vi "MKS_VIs.vi"() -> ()   [LabVIEW 2013]
uses:
  <userlib>/_mks/common/mks setpoint type.ctl
  <userlib>/_mks/common/mks alt status setpoint selection.ctl
  <userlib>/_mks/common/mks valve mode.ctl
  <userlib>/_mks/additional/mks request gain A (46).vi
  <userlib>/_mks/additional/mks request lead A value (41).vi
  <userlib>/_mks/additional/mks request analog setpoint type (25).vi
  <userlib>/_mks/additional/mks request setpoint analog value (0).vi
  <userlib>/_mks/additional/mks request softstart rate analog value (20).vi
  <userlib>/_mks/additional/mks request low threshold 1 (11).vi
panel:
  in  "stop":bool
  in  "valve mode":T1
  in  "setpoint value":dbl min=0.0 max=100.0 format="%.2g"
  in  "setpoint type":T2
  in  "setpoint selection":T3=enum."setpoint A"
  out "setpoint":dbl format="%.3g"
  out "setpoint type":T2
  out "error out":errorcluster
  out "Pressure (Torr)":dbl
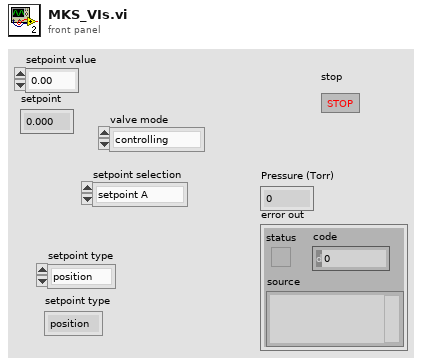
[diagram p1: front panel]
types:
  T1 = typedef "mks valve mode.ctl" = enum16{"controlling", "hold", "valve open", "unknoen", "valve close"}
  T2 = typedef "mks setpoint type.ctl" = enum16{"position", "pressure"}
  T3 = typedef "mks alt status setpoint selection.ctl" = enum16{"analog setpoint", "setpoint A", "setpoint B", "setpoint C", "setpoint D", "setpoint E"}
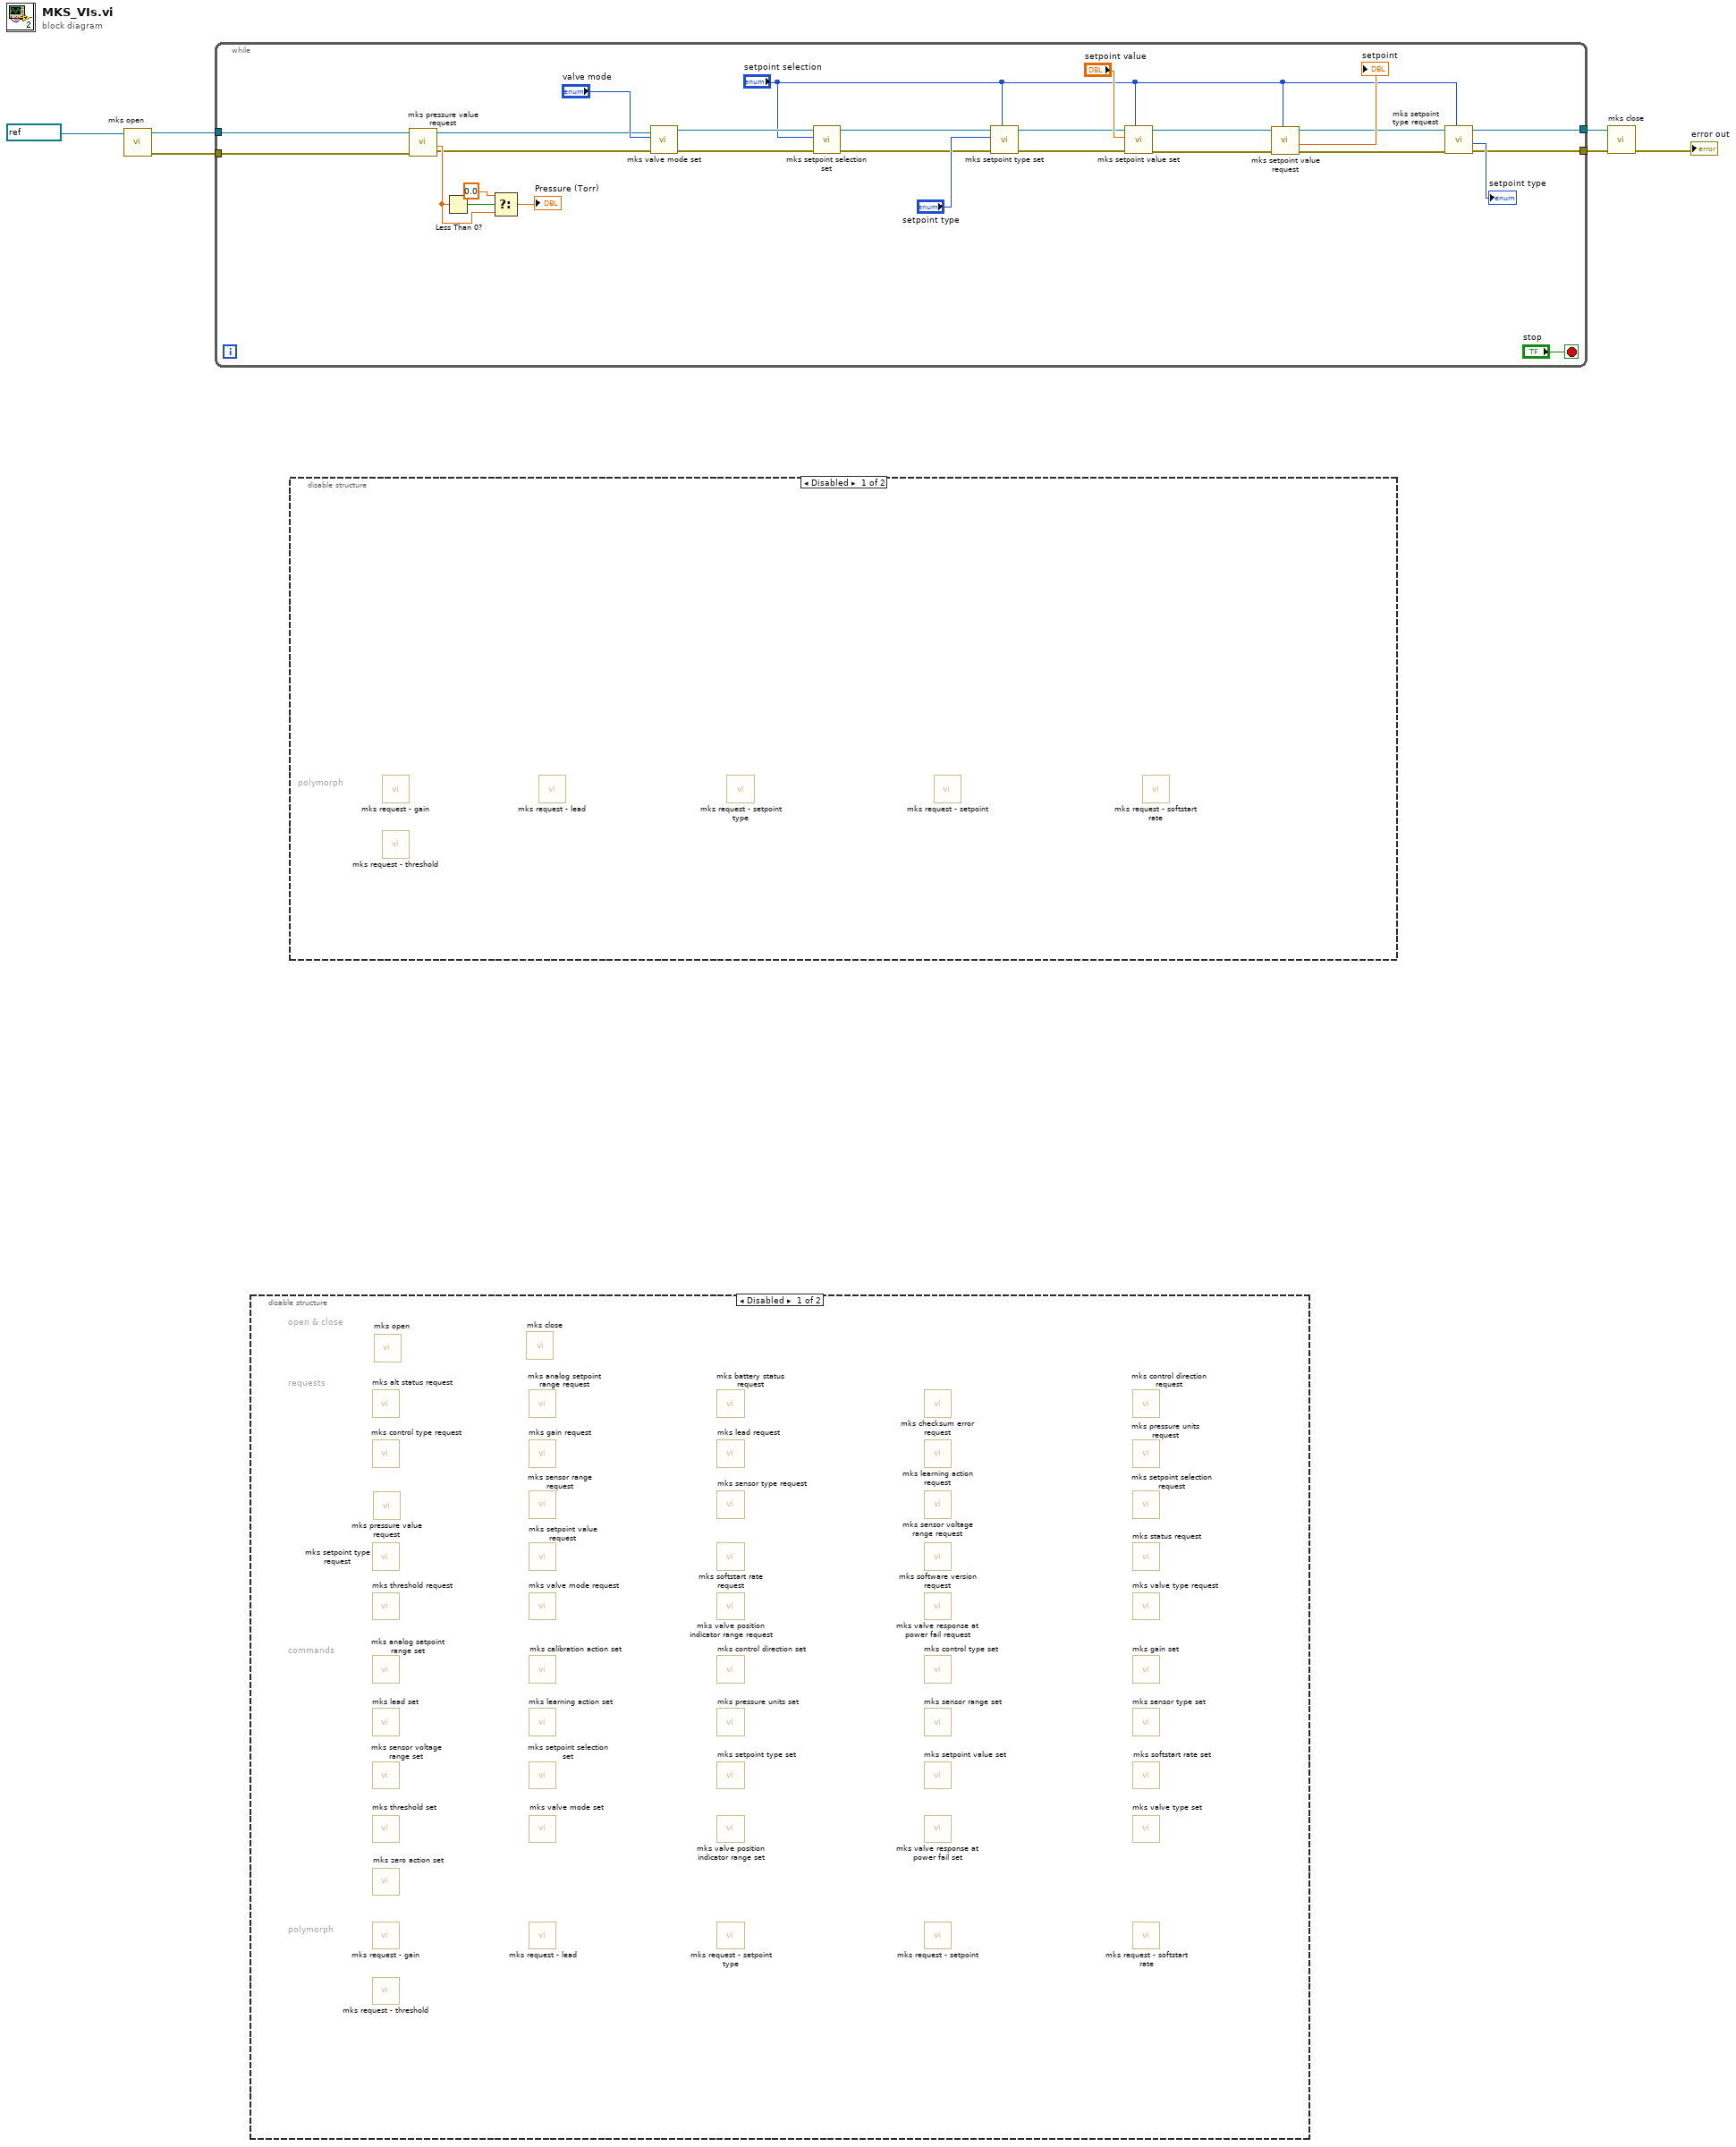
[diagram p0: block diagram]
diagram:
  n1 = call <userlib>:"mks open.vi"("VISA in"=refnum<visa-resource-name> "COM5") -> ("error out"=w6:errorcluster, "VISA out"=w5:refnum<visa-resource-name>)  [unwired: 9 in]
  n2 = while {
    tunnel: w6 -> [w33]
    tunnel: w5 -> [w32]
    tunnel: [w12] -> w2
    tunnel: [w11] -> w1
    stop <- "stop" stop-if-true
    n3 = call <userlib>:"mks pressure value request.vi"("error in (no error)"=w33, "VISA in"=w32) -> ("error out"=w9:errorcluster, "pressure"=w23:dbl, "VISA out"=w10:refnum<visa-resource-name>)  [unwired: 7 in]
    n4 = Less Than 0?(x=w23) -> (x < 0?=w31:bool)
    n5 = Select(t=0.0, s=w31, f=w23) -> (s? t:f=→"Pressure (Torr)":dbl)
    n6 = call <userlib>:"mks valve mode set.vi"("error in (no error)"=w9, "valve mode"="valve mode", "VISA in"=w10) -> ("error out"=w15:errorcluster, "VISA out"=w16:refnum<visa-resource-name>)  [unwired: 7 in]
    n7 = call <userlib>:"mks setpoint selection set.vi"("error in (no error)"=w15, "setpoint selection"="setpoint selection", "VISA in"=w16) -> ("error out"=w21:errorcluster, "VISA out"=w22:refnum<visa-resource-name>)  [unwired: 7 in]
    n8 = call <userlib>:"mks setpoint type set.vi"("setpoint selection"="setpoint selection", "error in (no error)"=w21, "setpoint type"="setpoint type", "VISA in"=w22) -> ("error out"=w19:errorcluster, "VISA out"=w20:refnum<visa-resource-name>)  [unwired: 6 in]
    n9 = call <userlib>:"mks setpoint value set.vi"("setpoint selection"="setpoint selection", "error in (no error)"=w19, "setpoint"="setpoint value", "VISA in"=w20) -> ("error out"=w17:errorcluster, "VISA out"=w18:refnum<visa-resource-name>)  [unwired: 6 in]
    n10 = call <userlib>:"mks setpoint value request.vi"("setpoint selection"="setpoint selection", "error in (no error)"=w17, "VISA in"=w18) -> ("error out"=w13:errorcluster, "setpoint"=→"setpoint":dbl, "VISA out"=w14:refnum<visa-resource-name>)  [unwired: 6 in]
    n11 = call <userlib>:"mks setpoint type request.vi"("setpoint selection"="setpoint selection", "error in (no error)"=w13, "VISA in"=w14) -> ("error out"=w12:errorcluster, "setpoint type"=→"setpoint type":T2, "VISA out"=w11:refnum<visa-resource-name>)  [unwired: 6 in]
  }
  n12 = disable-structure shown="Disabled" {
    frame Disabled {
      # "polymorph"
      # "commands"
      # "requests"
      # "open & close"
      n13 = call <userlib>:"mks alt status request.vi"() -> ()  [unwired: 9 in, 3 out]
      n14 = call <userlib>:"mks control type request.vi"() -> ()  [unwired: 9 in, 3 out]
      n15 = call <userlib>:"mks setpoint type request.vi"() -> ()  [unwired: 9 in, 3 out]
      n16 = call <userlib>:"mks threshold request.vi"() -> ()  [unwired: 9 in, 3 out]
      n17 = call <userlib>:"mks analog setpoint range set.vi"() -> ()  [unwired: 10 in, 2 out]
      n18 = call <userlib>:"mks lead set.vi"() -> ()  [unwired: 10 in, 2 out]
      n19 = call <userlib>:"mks sensor voltage range set.vi"() -> ()  [unwired: 10 in, 2 out]
      n20 = call <userlib>:"mks threshold set.vi"() -> ()  [unwired: 10 in, 2 out]
      n21 = call <userlib>:"mks zero action set.vi"() -> ()  [unwired: 10 in, 2 out]
      n22 = call-poly <userlib>:"mks request - gain.vi"() -> ()  [unwired: 9 in, 3 out]
      n23 = call-poly <userlib>:"mks request - threshold.vi"() -> ()  [unwired: 9 in, 3 out]
      n24 = call <userlib>:"mks pressure value request.vi"() -> ()  [unwired: 9 in, 3 out]
      n25 = call <userlib>:"mks open.vi"() -> ()  [unwired: 10 in, 2 out]
      n26 = call <userlib>:"mks close.vi"() -> ()  [unwired: 11 in, 1 out]
      n27 = call <userlib>:"mks analog setpoint range request.vi"() -> ()  [unwired: 9 in, 3 out]
      n28 = call <userlib>:"mks gain request.vi"() -> ()  [unwired: 9 in, 3 out]
      n29 = call <userlib>:"mks sensor range request.vi"() -> ()  [unwired: 9 in, 3 out]
      n30 = call <userlib>:"mks setpoint value request.vi"() -> ()  [unwired: 9 in, 3 out]
      n31 = call <userlib>:"mks valve mode request.vi"() -> ()  [unwired: 9 in, 3 out]
      n32 = call <userlib>:"mks calibration action set.vi"() -> ()  [unwired: 10 in, 2 out]
      n33 = call <userlib>:"mks learning action set.vi"() -> ()  [unwired: 10 in, 2 out]
      n34 = call <userlib>:"mks setpoint selection set.vi"() -> ()  [unwired: 10 in, 2 out]
      n35 = call <userlib>:"mks valve mode set.vi"() -> ()  [unwired: 10 in, 2 out]
      n36 = call-poly <userlib>:"mks request - lead.vi"() -> ()  [unwired: 9 in, 3 out]
      n37 = call <userlib>:"mks battery status request.vi"() -> ()  [unwired: 9 in, 3 out]
      n38 = call <userlib>:"mks lead request.vi"() -> ()  [unwired: 9 in, 3 out]
      n39 = call <userlib>:"mks sensor type request.vi"() -> ()  [unwired: 9 in, 3 out]
      n40 = call <userlib>:"mks softstart rate request.vi"() -> ()  [unwired: 9 in, 3 out]
      n41 = call <userlib>:"mks valve position indicator range request.vi"() -> ()  [unwired: 9 in, 3 out]
      n42 = call <userlib>:"mks control direction set.vi"() -> ()  [unwired: 10 in, 2 out]
      n43 = call <userlib>:"mks pressure units set.vi"() -> ()  [unwired: 10 in, 2 out]
      n44 = call <userlib>:"mks setpoint type set.vi"() -> ()  [unwired: 10 in, 2 out]
      n45 = call <userlib>:"mks valve position indicator range set.vi"() -> ()  [unwired: 10 in, 2 out]
      n46 = call-poly <userlib>:"mks request - setpoint type.vi"() -> ()  [unwired: 9 in, 3 out]
      n47 = call <userlib>:"mks checksum error request.vi"() -> ()  [unwired: 9 in, 3 out]
      n48 = call <userlib>:"mks learning action request.vi"() -> ()  [unwired: 9 in, 3 out]
      n49 = call <userlib>:"mks sensor voltage range request.vi"() -> ()  [unwired: 9 in, 3 out]
      n50 = call <userlib>:"mks software version request.vi"() -> ()  [unwired: 9 in, 3 out]
      n51 = call <userlib>:"mks valve response at power fail request.vi"() -> ()  [unwired: 9 in, 3 out]
      n52 = call <userlib>:"mks control type set.vi"() -> ()  [unwired: 10 in, 2 out]
      n53 = call <userlib>:"mks sensor range set.vi"() -> ()  [unwired: 10 in, 2 out]
      n54 = call <userlib>:"mks setpoint value set.vi"() -> ()  [unwired: 10 in, 2 out]
      n55 = call <userlib>:"mks valve response at power fail set.vi"() -> ()  [unwired: 10 in, 2 out]
      n56 = call-poly <userlib>:"mks request - setpoint.vi"() -> ()  [unwired: 9 in, 3 out]
      n57 = call <userlib>:"mks control direction request.vi"() -> ()  [unwired: 9 in, 3 out]
      n58 = call <userlib>:"mks pressure units request.vi"() -> ()  [unwired: 9 in, 3 out]
      n59 = call <userlib>:"mks setpoint selection request.vi"() -> ()  [unwired: 9 in, 3 out]
      n60 = call <userlib>:"mks status request.vi"() -> ()  [unwired: 9 in, 3 out]
      n61 = call <userlib>:"mks valve type request.vi"() -> ()  [unwired: 9 in, 3 out]
      n62 = call <userlib>:"mks gain set.vi"() -> ()  [unwired: 10 in, 2 out]
      n63 = call <userlib>:"mks sensor type set.vi"() -> ()  [unwired: 10 in, 2 out]
      n64 = call <userlib>:"mks softstart rate set.vi"() -> ()  [unwired: 10 in, 2 out]
      n65 = call <userlib>:"mks valve type set.vi"() -> ()  [unwired: 10 in, 2 out]
      n66 = call-poly <userlib>:"mks request - softstart rate.vi"() -> ()  [unwired: 9 in, 3 out]
    }
    frame Enabled {
    }
  }
  n67 = disable-structure shown="Disabled" {
    frame Disabled {
      # "polymorph"
      n68 = call-poly <userlib>:"mks request - gain.vi"() -> ()  [unwired: 9 in, 3 out]
      n69 = call-poly <userlib>:"mks request - threshold.vi"() -> ()  [unwired: 9 in, 3 out]
      n70 = call-poly <userlib>:"mks request - lead.vi"() -> ()  [unwired: 9 in, 3 out]
      n71 = call-poly <userlib>:"mks request - setpoint type.vi"() -> ()  [unwired: 9 in, 3 out]
      n72 = call-poly <userlib>:"mks request - setpoint.vi"() -> ()  [unwired: 9 in, 3 out]
      n73 = call-poly <userlib>:"mks request - softstart rate.vi"() -> ()  [unwired: 9 in, 3 out]
    }
    frame Enabled {
    }
  }
  n74 = call <userlib>:"mks close.vi"("error in (no error)"=w2, "VISA in"=w1) -> ("error out"=→"error out":errorcluster)  [unwired: 9 in]
